vi "Launcher.vi"   [LabVIEW 2020]
uses:
  First Actor/First Actor/First Actor.lvclass
  C:/Program Files (x86)/National Instruments/LabVIEW 2020/vi.lib/ActorFramework/Actor/Actor.lvclass
  First Actor/First Actor Messages/PopUp Msg/PopUp Msg.lvclass/PopUp Msg.ctl
  <vilib>/ActorFramework/Message Enqueuer/Message Enqueuer.lvclass/Message Enqueuer.ctl
  <vilib>/ActorFramework/Message Enqueuer/Enqueue.vi
  First Actor/First Actor Messages/PopUp Msg/PopUp Msg.lvclass
  C:/Program Files (x86)/National Instruments/LabVIEW 2020/vi.lib/ActorFramework/Message/Message.lvclass
  <vilib>/ActorFramework/Stop Msg/Stop Msg.lvclass
  <vilib>/ActorFramework/Message Priority Queue/Priority Enqueue.vi
  <vilib>/ActorFramework/Actor/Actor.lvclass
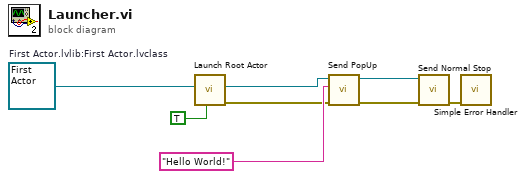
[diagram p0: block diagram]
diagram:
  w8 = refnum<class "First Actor.lvclass"> refnum  # First Actor.lvlib:First Actor.lvclass
  n1 = call <vilib>:"Launch Root Actor.vi"("Open Actor Core front panel? (F)"=TRUE, "Actor"=w8) -> ("error out"=w2:errorcluster, "Actor's Enqueuer"=w7:refnum<class "Message Enqueuer.lvclass">)  [unwired: 8 in]
  n2 = call "Send PopUp.vi"("error in (no error)"=w2, "Text"="Hello World!", "Message Enqueuer"=w7) -> ("error out"=w3:errorcluster, "Message Enqueuer out"=w5:refnum<class "Message Enqueuer.lvclass">)  [unwired: 7 in]
  n3 = call <vilib>:"Send Normal Stop.vi"("error in (no error)"=w3, "Message Enqueuer"=w5) -> ("error out"=w4:errorcluster)  [unwired: 9 in]
  n4 = call <vilib>:"Simple Error Handler.vi"("error in (no error)"=w4) -> ()  [unwired: 4 in, 5 out]
